vi "2084远程反控参数运行间隔解析.vi"(11 "字符串":string="PolId=w01018,RunInterval=4;PolId=w01019,RunInterval=4;") -> (2 "Value":string[](array[string]), 3 "因子编码":string[](array[string]))   [LabVIEW 2016, in "数据传输系统-05.lvlib"]
uses:
  <vilib>/regexp/Match Regular Expression.xnode
panel:
  out "数组":string[](array[string])
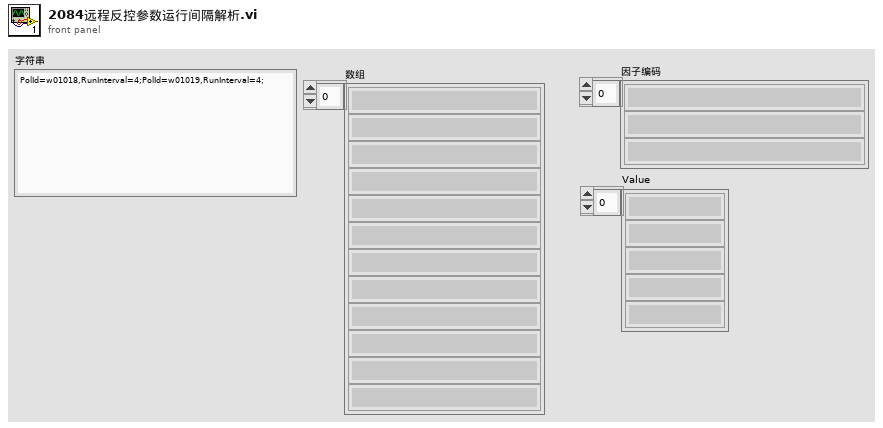
[diagram p1: front panel]
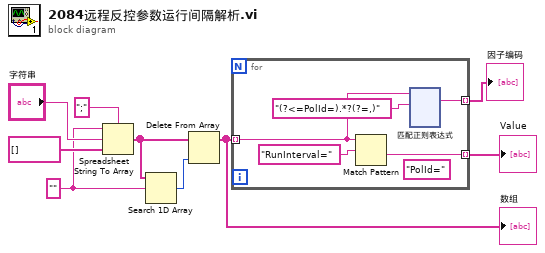
[diagram p0: block diagram]
diagram:
  w4 = ""
  n1 = Spreadsheet String To Array(delimiter (Tab)=";" ("分隔符(Tab)"), format string=w4, spreadsheet string="字符串", array type (2D Dbl)=string[] []) -> (array=w3:string[])
  n2 = Search 1D Array(1D array=w3, element=w4) -> (index of element=w2:i32)  [unwired: 1 in]
  n3 = Delete From Array(array=w3, index=w2) -> (array with subset deleted=w1:string[])  [unwired: 1 in, 1 out]
  "数组" <- w1
  n4 = for {
    tunnel: w1 -> [w12] mode=indexing
    tunnel: [w13] -> w5 mode=indexing
    tunnel: [w11] -> w6 mode=indexing
    (unwired) "PolId=" ("正则表达式")
    n5 = Match Pattern(string=w12, regular expression="RunInterval=" ("正则表达式")) -> (after substring=w13:string)  [unwired: 1 in, 3 out]
    n6 = xnode "匹配正则表达式"("输入字符串"=w12, "正则表达式"="(?<=PolId=).*?(?=,)") -> ("所有匹配"=w11:string)  [unwired: 4 in, 4 out]
  }
  "因子编码" <- w6
  "Value" <- w5
